vi "_PC_Turbo_ClusterItemsString.vi"(8 "error in (no error)":errorcluster, 10 "JSON string":string) -> (0 "error out":errorcluster, 2 "result string":string)   [LabVIEW 2018]
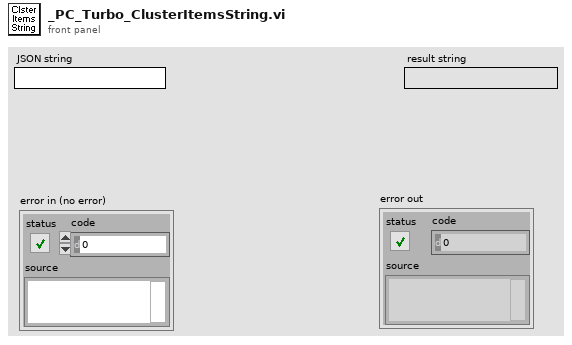
[diagram p1: front panel]
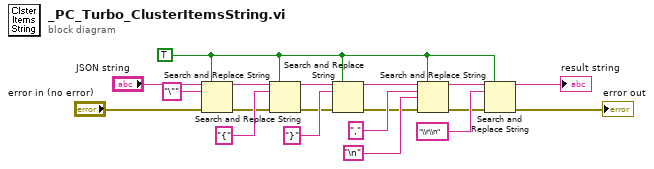
[diagram p0: block diagram]
diagram:
  w7 = TRUE ("replace all? (F)")
  n1 = Search and Replace String(replace all?=w7, input string="JSON string", search string="\"", error in="error in (no error)") -> (result string=w17:string, error out=w4:errorcluster)  [unwired: 4 in, 2 out]
  n2 = Search and Replace String(replace all?=w7, input string=w17, search string="{" ("input string"), error in=w4) -> (result string=w15:string, error out=w3:errorcluster)  [unwired: 4 in, 2 out]
  n3 = Search and Replace String(replace all?=w7, input string=w15, search string="}" ("input string"), error in=w3) -> (result string=w14:string, error out=w2:errorcluster)  [unwired: 4 in, 2 out]
  n4 = Search and Replace String(replace all?=w7, input string=w14, search string="," ("input string"), replace string="\n", error in=w2) -> (result string=w10:string, error out=w1:errorcluster)  [unwired: 3 in, 2 out]
  n5 = Search and Replace String(replace all?=w7, input string=w10, search string="\\r\\n", error in=w1) -> (result string=→"result string":string, error out=→"error out":errorcluster)  [unwired: 4 in, 2 out]
